vi "findSumm.vi"(10 "#in":i32, 11 "body in in":string) -> (3 "body out":string)   [LabVIEW 2013]
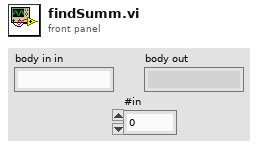
[diagram p1: front panel]
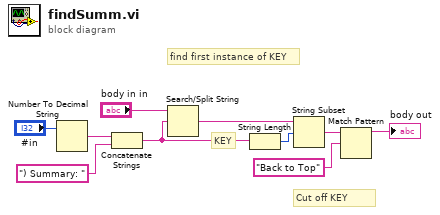
[diagram p0: block diagram]
diagram:
  # "Cut off KEY"
  # "KEY"
  # "find first instance of KEY"
  n1 = Number To Decimal String(number="#in") -> (decimal integer string=w1:string)  [unwired: 1 in]
  n2 = Concatenate Strings(w1, ") Summary: " ("KEY")) -> (w4:string)
  n3 = Search/Split String(string="body in in", search string/char (-)=w4) -> (match + rest of string=w8:string)  [unwired: 1 in, 2 out]
  n4 = String Length(string=w4) -> (length=w9:i32)
  n5 = String Subset(string=w8, offset (0)=w9) -> (substring=w6:string)  [unwired: 1 in]
  n6 = Match Pattern(string=w6, regular expression="Back to Top") -> (before substring=→"body out":string)  [unwired: 1 in, 3 out]
